vi "BK Precision 5490C Series Acquire Multiple.vi"() -> ()   [LabVIEW 2018]
doc: "This example shows how to setup and acquire multiple measurements."
uses:
  <instrlib>/BK Precision 5490C Series/Public/Data/Read (Multiple Points).vi
  <instrlib>/BK Precision 5490C Series/BK Precision 5490C Series.lvlib
panel:
  in  "Measurement Function (0: Voltage DC)":i32(ring) items=["Voltage DC", "Voltage DC Ratio", "Voltage AC", "Current DC", "Current AC", "Resistance 2-Wire", "Resistance 4-Wire", "Frequency", "Period", "Capacitance", "Continuity", "Diode", "Temperature"]
  in  "Sample Count (10)":i32=10
  out "Measurements":dbl[](array[numeric])
  in  "Wait Time (200 ms)":u32=200
  in  "VISA resource name":refnum<visa-resource-name>
  # "(c) 2020 B&K Precision Corporation.  ALL RIGHTS RESERVED."
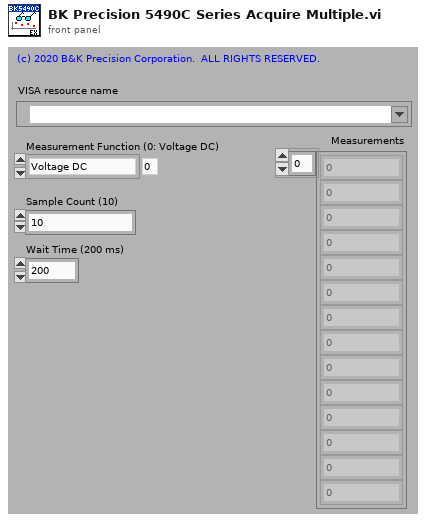
[diagram p1: front panel]
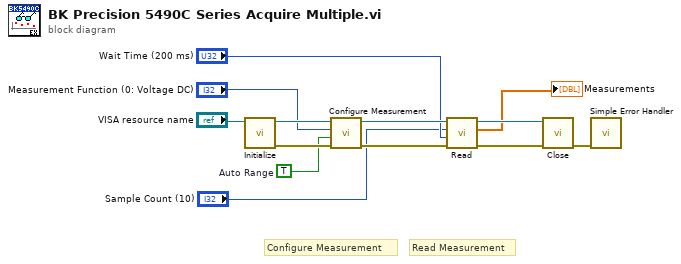
[diagram p0: block diagram]
diagram:
  w10 = TRUE  # Auto Range
  # "Read Measurement"
  # "Configure Measurement"
  n1 = call <instrlib>:"Initialize.vi"("VISA resource name"="VISA resource name") -> ("error out"=w11:errorcluster, "VISA resource name out"=w12:refnum<visa-resource-name>)  [unwired: 4 in, 5 out]
  n2 = call <instrlib>:"Configure Measurement.vi"("error in (no error)"=w11, "Auto Range (T: Enable)"=w10, "Measurement Function (0: Voltage DC)"="Measurement Function (0: Voltage DC)", "VISA resource name"=w12) -> ("error out"=w8:errorcluster, "VISA resource name out"=w7:refnum<visa-resource-name>)  [unwired: 1 in, 5 out]
  n3 = call-poly <instrlib>:"Read.vi"("error in (no error)"=w8, "Timeout (10000 ms)"="Wait Time (200 ms)", "Sample Count (10)"="Sample Count (10)", "VISA resource name"=w7) -> ("error out"=w9:errorcluster, "Measurements"=→"Measurements":dbl[], "VISA resource name out"=w6:refnum<visa-resource-name>)  [unwired: 5 out]
  n4 = call <instrlib>:"Close.vi"("error in (no error)"=w9, "VISA resource name"=w6) -> ("error out"=w13:errorcluster)  [unwired: 9 out]
  n5 = call <vilib>:"Simple Error Handler.vi"("error in (no error)"=w13) -> ()  [unwired: 1 in, 8 out]
